vi "select ROI.vi"(8 "error in (no error)":errorcluster, 11 "Thorcam in":refnum<class "Thorcam.lvclass">) -> (0 "error out":errorcluster, 3 "Thorcam out":refnum<class "Thorcam.lvclass">)   [LabVIEW 2012, in "Thorcam.lvclass"]
uses:
  Thorcam.lvclass
  Thorcam.lvclass/Thorcam.ctl
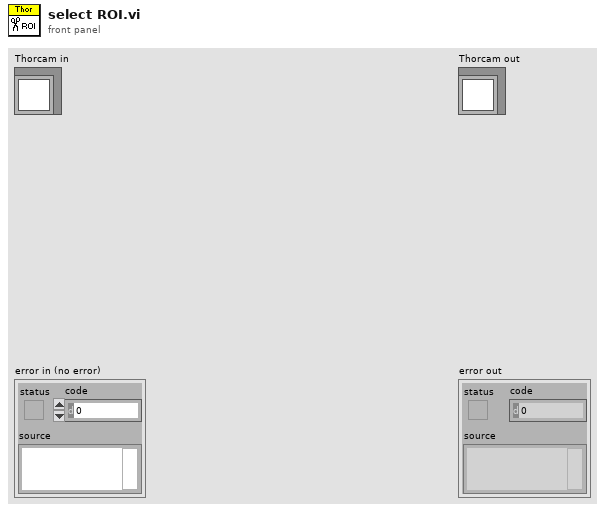
[diagram p1: front panel]
types:
  T1 = typedef "IMAQ Image.ctl" = refnum<image>
  T2 = typedef "ROI Descriptor" = cluster{"Global Rectangle":i32[], "Contours":cluster{"ID":enum32{"External", "Internal"}, "Type":u32, "Coordinates":i32[]}[]}
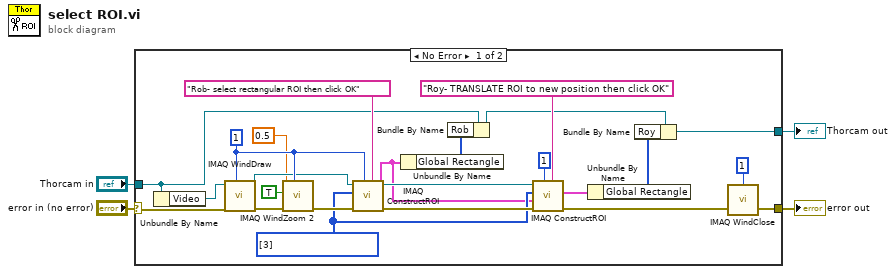
[diagram p0: block diagram]
diagram:
  n1 = case shown="No Error" "error in (no error)" {
    selector: "error in (no error)" -> [w8 w30]
    tunnel: [w10 w30] -> w4
    tunnel: [w19 w29] -> w2
    tunnel: "Thorcam in" -> [w7 w29]
    frame No Error {
      w15 = 1 ("Window Number (0...15)")
      w13 = u32[] [3] items=["No Selection", "Point", "Line", "Rectangle", "Oval", "Polygon", "Freehand Region", "Annulus", "Zoom", "Pan", "Broken Line", "Freehand Line", "Rotated Rectangle"] ("Tools")
      n2 = Unbundle By Name(w7) -> ("Video"=w6:T1)
      n3 = call "IMAQ WindDraw"("Window Number (0...15)"=w15, "error in (no error)"=w8, "Image"=w6) -> ("error out"=w18:errorcluster, "Image Out (duplicate)"=w14:T1)  [unwired: 7 in]
      n4 = call "IMAQ WindZoom 2"("Window Number (0...15)"=w15, "error in (no error)"=w18, "Zoom to Fit? (False)"=TRUE, "Zoom Factor"=sgl 0.5) -> ("error out"=w17:errorcluster)  [unwired: 4 in, 3 out]
      n5 = call "IMAQ ConstructROI"("Prompt"="Rob- select rectangular ROI then click OK", "Window Number (-1...15)"=w15, "error in (no error)"=w17, "Tools"=w13, "Image"=w14) -> ("error out"=w27:errorcluster, "ROI Descriptor Out"=w12:T2, "Image Out (duplicate)"=w26:T1)  [unwired: 3 in, 1 out]
      n6 = Unbundle By Name(w12) -> ("Global Rectangle"=w28:i32[])
      n7 = Bundle By Name(cluster=w7, "Rob"=w28) -> (w20:refnum<class "Thorcam.lvclass">)
      n8 = call "IMAQ ConstructROI"("Prompt"="Roy- TRANSLATE ROI to new position then click OK", "Window Number (-1...15)"=1, "error in (no error)"=w27, "ROI Descriptor In (None)"=w12, "Tools"=w13, "Image"=w26) -> ("error out"=w11:errorcluster, "ROI Descriptor Out"=w22:T2)  [unwired: 2 in, 2 out]
      n9 = Unbundle By Name(w22) -> ("Global Rectangle"=w21:i32[])
      n10 = Bundle By Name(cluster=w20, "Roy"=w21) -> (w19:refnum<class "Thorcam.lvclass">)
      n11 = call "IMAQ WindClose"("Window Number (0...15)"=1, "error in (no error)"=w11) -> ("error out"=w10:errorcluster)  [unwired: 4 in]
    }
    frame Error {
    }
  }
  "error out" <- w4
  "Thorcam out" <- w2
